vi "Set_Local_Origin.vi"(0 "PortNumber":u8=7) -> (1 "Received String1":string, 2 "Received String2":string, 3 "OK Done":bool)   [LabVIEW 2013]
panel:
  out "Received String1 2":string
  in  "PortNumber 2":u8=8
  out "OK Done 2":bool
  out "Received String2 2":string
  # "Port Number 0=COM1"
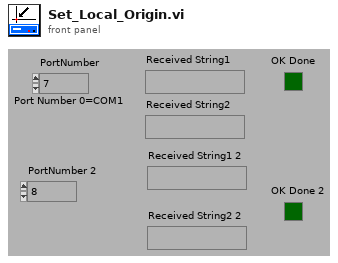
[diagram p1: front panel]
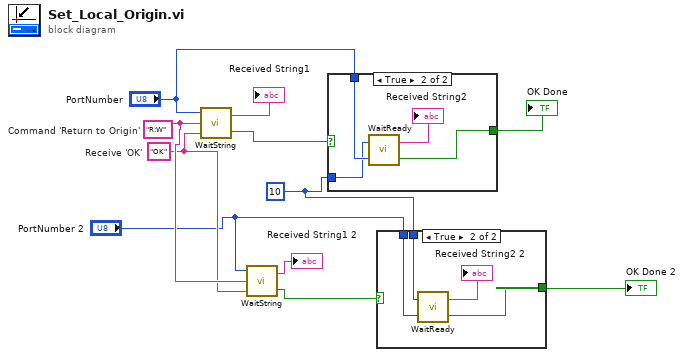
[diagram p0: block diagram]
diagram:
  w6 = 10
  w4 = "OK"  # Receive 'OK'
  w5 = "R:W"  # Command 'Return to Origin'
  n1 = call "WaitString.vi"("String to Receive"=w4, "String to Send"=w5, "PortNumber"="PortNumber") -> ("OK Done"=w8:bool, "String Received"=→"Received String1":string)
  n2 = call "WaitString.vi"("String to Receive"=w4, "String to Send"=w5, "PortNumber"="PortNumber 2") -> ("OK Done"=w1:bool, "String Received"=→"Received String1 2":string)
  n3 = case shown="True" w8 {
    selector: w8 -> [w12 _]
    tunnel: "PortNumber" -> [_ w16]
    tunnel: [w12 w14] -> w11
    tunnel: w6 -> [_ w13]
    frame False {
    }
    frame True {
      n4 = call "WaitReady.vi"("PortNumber"=w16, "Residence time in ms"=w13) -> ("OK Done"=w14:bool, "String Received"=→"Received String2":string)
    }
  }
  "OK Done" <- w11
  n5 = case shown="True" w1 {
    selector: w1 -> [w17 _]
    tunnel: "PortNumber 2" -> [_ w21]
    tunnel: [w17 w19] -> w7
    tunnel: w6 -> [_ w18]
    frame False {
    }
    frame True {
      n6 = call "WaitReady.vi"("PortNumber"=w21, "Residence time in ms"=w18) -> ("OK Done"=w19:bool, "String Received"=→"Received String2 2":string)
    }
  }
  "OK Done 2" <- w7
